vi "DumpTest.vi"() -> ()   [LabVIEW 2009]
uses:
  Packet.ctl
panel:
  out "ReceivedBytes":T1[](array[typedef])
  in  "VISA resource In":refnum<visa-resource-name>
  in  "error In":errorcluster
  out "error out":errorcluster
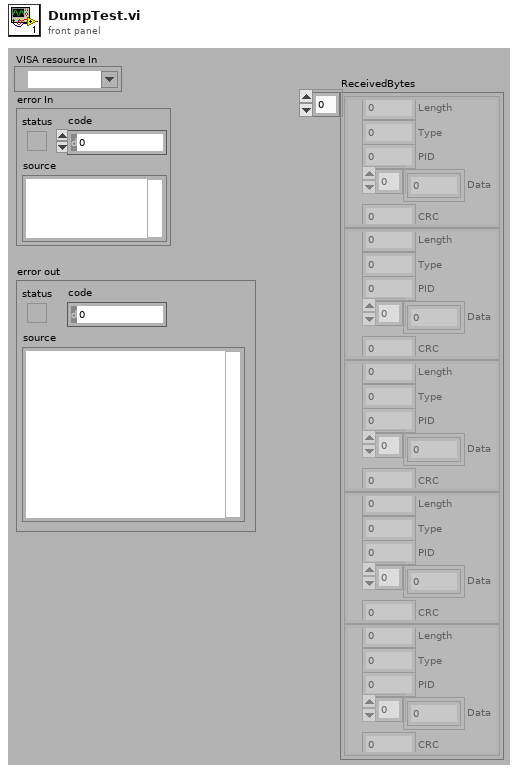
[diagram p1: front panel]
types:
  T1 = typedef "Packet.ctl" = cluster{"Length":u8, "Type":u8, "PID":u8, "Data":u8[], "CRC":u8}
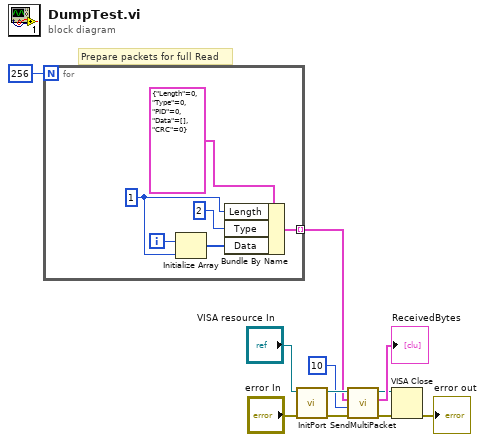
[diagram p0: block diagram]
diagram:
  # "Prepare packets for full Read"
  n1 = for {
    N: 256 -> [_]
    tunnel: [w15] -> w6 mode=indexing
    i -> [w14]
    w12 = 1 ("dimension size")
    n2 = Initialize Array(w14, w12) -> (w13:i32[])
    n3 = Bundle By Name(cluster=T1 {"Length"=0, "Type"=0, "PID"=0, "Data"=[], "CRC"=0} ("Transmit"), "Length"=w12, "Type"=u8 2, "Data"=w13) -> (w15:T1)
  }
  n4 = call "InitPort.vi"("error in (no error)"="error In", "VISA resource name"="VISA resource In") -> ("error out"=w4:errorcluster, "VISA resource name out"=w7:refnum<visa-resource-name>)  [unwired: 8 in]
  n5 = call "SendMultiPacket.vi"("error in (no error)"=w4, "PIDIn"=u8 10, "Packets In"=w6, "VISA resource name"=w7) -> ("error out"=w2:errorcluster, "ReceivedBytes"=→"ReceivedBytes":T1[], "VISA resource name out"=w3:refnum<visa-resource-name>)  [unwired: 4 in, 1 out]
  n6 = VISA Close(VISA resource name=w3, error in (no error)=w2) -> (error out=→"error out":errorcluster)
